vi "finishTopicSection.vi"(8 "error in (no error)":errorcluster, 11 "Module in":refnum<class "Module.lvclass">) -> (0 "error out":errorcluster, 2 "reachedEnd?":bool, 3 "Module out":refnum<class "Module.lvclass">)   [LabVIEW 2015, in "Module.lvclass"]
uses:
  Module.lvclass
  Module.lvclass/Module.ctl
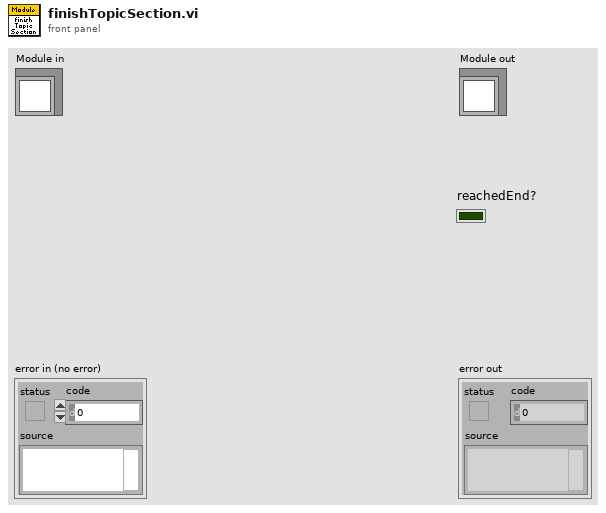
[diagram p1: front panel]
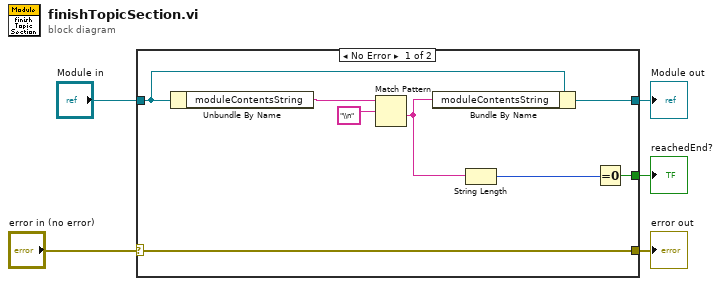
[diagram p0: block diagram]
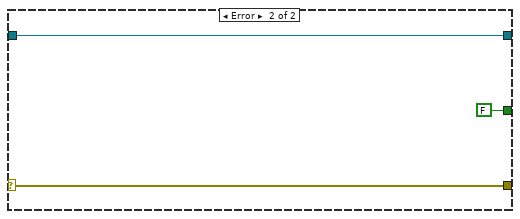
[diagram p2: hidden frame]
diagram:
  n1 = case shown="No Error" "error in (no error)" {
    selector: "error in (no error)" -> [w13 w16]
    tunnel: [w13 w16] -> w4
    tunnel: [w9 w15] -> w2
    tunnel: "Module in" -> [w10 w15]
    tunnel: [w11 FALSE] -> w1
    frame No Error {
      n2 = Unbundle By Name(w10) -> ("moduleContentsString"=w8:string)
      n3 = Match Pattern(string=w8, regular expression="\\n" ("string")) -> (after substring=w6:string)  [unwired: 1 in, 3 out]
      n4 = Bundle By Name(cluster=w10, "moduleContentsString"=w6) -> (w9:refnum<class "Module.lvclass">)
      n5 = String Length(string=w6) -> (length=w12:i32)
      n6 = Equal To 0?(x=w12) -> (x = 0?=w11:bool)
    }
    frame Error {
    }
  }
  "error out" <- w4
  "Module out" <- w2
  "reachedEnd?" <- w1
